vi "FdxCmdEDESubControlExCvi.vi"(6 "EDESubCntlExIn":T1, 8 "error in":errorcluster, 9 "EDESubCntlIn":T2, 10 "EDESubscriberHandle":u32, 11 "InstrumentHandle":u32) -> (0 "error out":errorcluster, 3 "InstrumentHandle":u32)   [LabVIEW 2020, in "AIM664LV.lvlib"]
doc: "This function is used to control the EDE subscriber. It provides extended functionality which allows the setting of the EDE Validation parameters."
uses:
  AIM664LV.lvlib
  AFDX_LibraryAdmin/FdxGlobalDllPath.vi
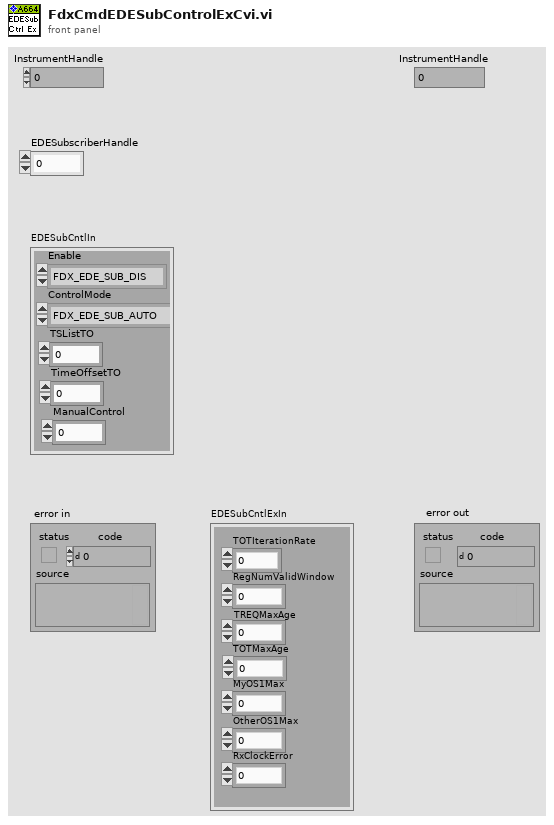
[diagram p1: front panel]
types:
  T1 = cluster{"TOTIterationRate":u32, "RegNumValidWindow":u32, "TREQMaxAge":u32, "TOTMaxAge":u32, "MyOS1Max":u32, "OtherOS1Max":u32, "RxClockError":u32}
  T2 = cluster{"Enable":enum32{"FDX_EDE_SUB_DIS", "FDX_EDE_SUB_ENA"}, "ControlMode":enum32{"FDX_EDE_SUB_AUTO"}, "TSListTO":u32, "TimeOffsetTO":u32, "ManualControl":u32}
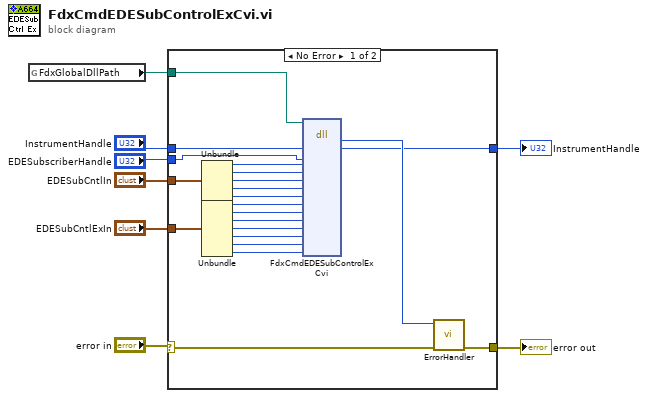
[diagram p0: block diagram]
diagram:
  n1 = global read "FdxGlobalDllPath.vi" "FdxGlobalDllPath"() -> (w6:path)
  n2 = case shown="No Error" "error in" {
    selector: "error in" -> [w28 w31]
    tunnel: [w29 w31] -> w8
    tunnel: w6 -> [w14 _]
    tunnel: [w13 w30] -> w5
    tunnel: "InstrumentHandle" -> [w12 w30]
    tunnel: "EDESubscriberHandle" -> [w11 _]
    tunnel: "EDESubCntlExIn" -> [w10 _]
    tunnel: "EDESubCntlIn" -> [w9 _]
    frame No Error {
      n3 = Unbundle(w9) -> ("Enable"=w20:enum32{"FDX_EDE_SUB_DIS", "FDX_EDE_SUB_ENA"}, "ControlMode"=w21:enum32{"FDX_EDE_SUB_AUTO"}, "TSListTO"=w22:u32, "TimeOffsetTO"=w19:u32, "ManualControl"=w18:u32)
      n4 = Unbundle(w10) -> ("TOTIterationRate"=w26:u32, "RegNumValidWindow"=w25:u32, "TREQMaxAge"=w24:u32, "TOTMaxAge"=w23:u32, "MyOS1Max"=w17:u32, "OtherOS1Max"=w16:u32, "RxClockError"=w15:u32)
      n5 = dll-call lib="aim_fdx.19.dll" fn="FdxCmdEDESubControlExCvi"(path in=w14, "InstrumentHandle"=w12, "EDESubscriberHandle"=w11, "Enable"=w20, "ControlMode"=w21, "TSListTO"=w22, "TimeOffsetTO"=w19, "ManualControl"=w18, "TOTiterationRate"=w26, "RegNumValidWindow"=w25, "TREQMaxAge"=w24, "TOTMaxAge"=w23, "MyOS1Max"=w17, "OtherOS1Max"=w16, "RxClockErrior"=w15) -> ("status"=w27:i32, "InstrumentHandle"=w13:u32)  [unwired: 13 in, 4 out]
      n6 = call "ErrorHandler.vi"("error in"=w28, "AIM Error"=w27) -> ("error out"=w29:errorcluster)  [unwired: 9 in]
    }
    frame Error {
    }
  }
  "error out" <- w8
  "InstrumentHandle" <- w5
